vi "Read Image on Button.vi"(4 "Save in temp directory?":bool=TRUE, 6 "Append Name?":bool, 9 "image item":i32, 11 "File with Button":path) -> (0 "error out":errorcluster, 3 "png file out":path)   [LabVIEW 2021]
doc: "This example VI was obtained from this post. This strips out the saving profile and just reads the image on an existing button.\n\nhttps://forums.ni.com/t5/LabVIEW-APIs-Discussions/Set-TRUE-FALSE-Image-of-a-boolean-control-automatically-using/m-p/3419083/highlight/true#M868\n\n<b>WARNING</b>\nThis VI uses a dll call to the resource file for a LabVIEW VI/CTL - it is searching the binary data for the PNG images that the VI or CTL contains\n\n<b>Code Developed By:</b>\nTechnology Service Corporation\n1983 S Liberty Drive\nBloomington, IN 47403\nPhone: 812 558-7100\nwww.tsc.com/atcs\n\nDeveloper:\nDaniel Coons"
panel:
  out "binary PNG Data":string
  out "Resources":string[](array[string])
  # "For DEBUG"
  # "MNGI resources are 6 images\non buttons (pressed, hover, etc)\n\n-When set to a \"decal\", it should\nbe the only one"
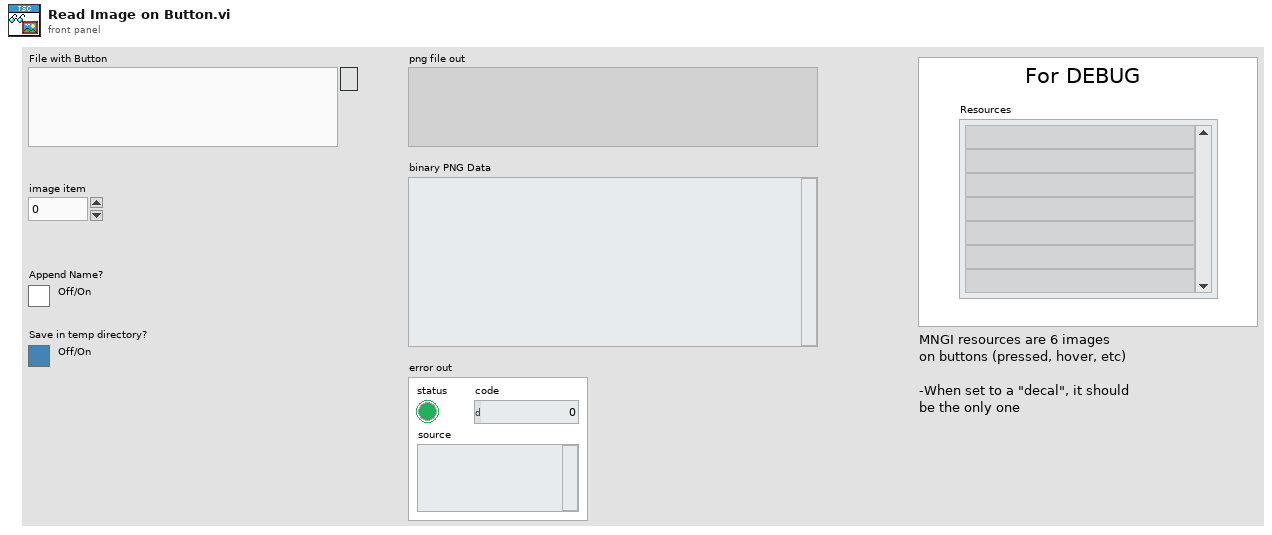
[diagram p1: front panel]
types:
  T1 = cluster{"type":u32, "id":i32, "name":string, "binary data":string}[]
  T2 = cluster{"type":u32, "id":i32, "name":string, "binary data":string}
  T3 = enum16{"open", "replace", "create", "open or create", "replace or create", "replace or create with confirmation"}
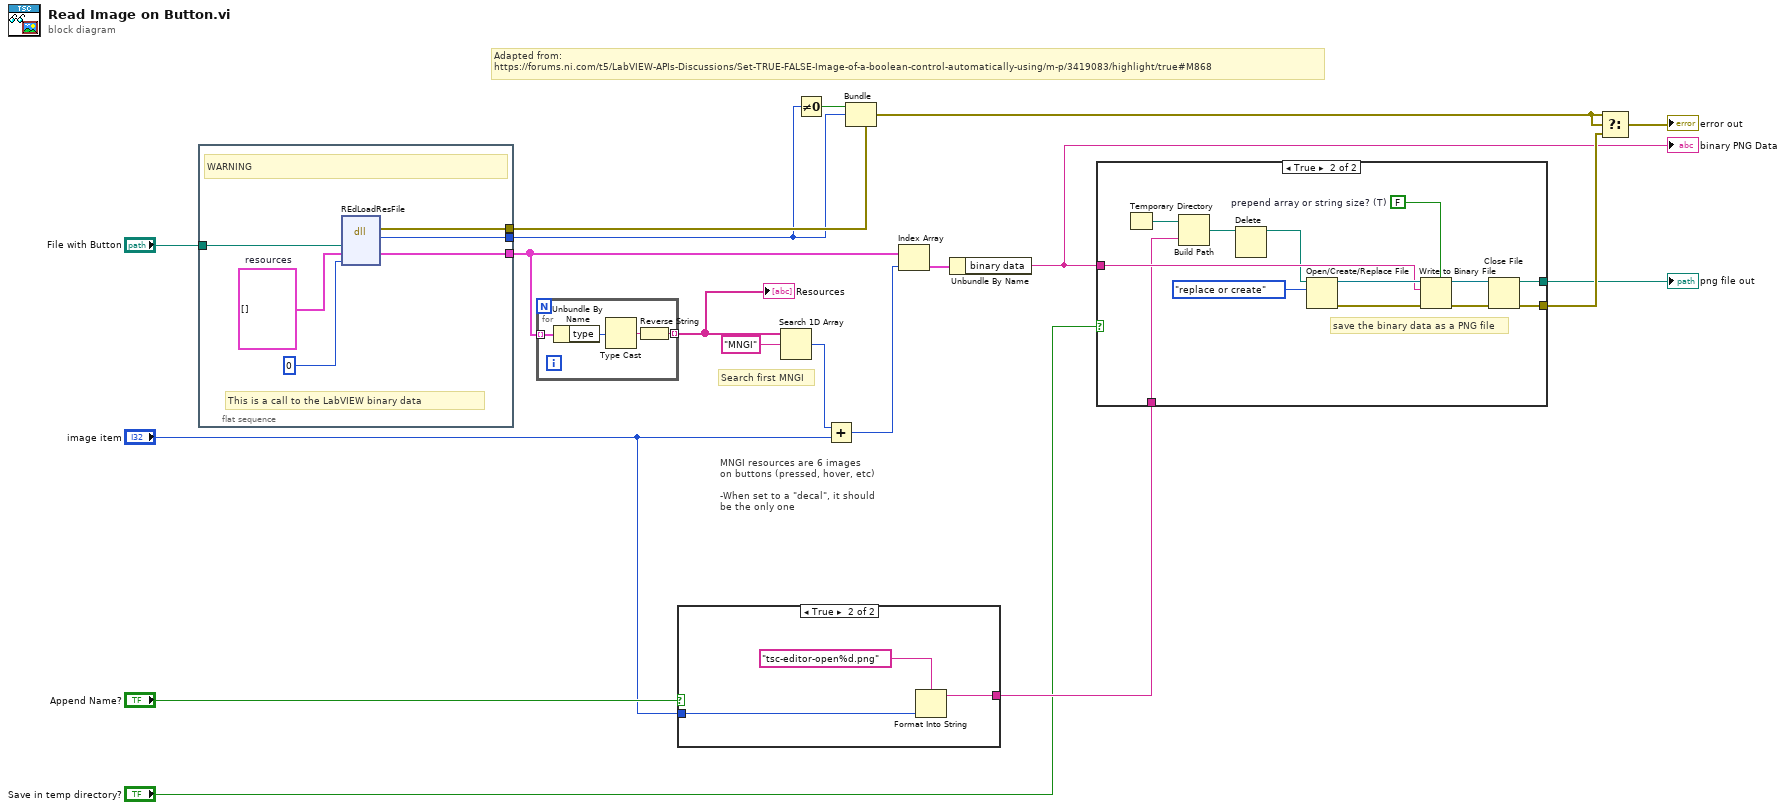
[diagram p0: block diagram]
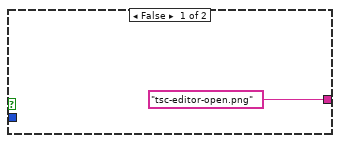
[diagram p3: hidden frame]
diagram:
  # "MNGI resources are 6 images\non buttons (pressed, hover, etc)\n\n-When set to a \"decal\", it should\nbe the only one"
  # "Adapted from:\nhttps://forums.ni.com/t5/LabVIEW-APIs-Discussions/Set-TRUE-FALSE-Image-of-a-boolean-control-automatically-using/m-p/3419083/highlight/true#M868"
  # "Search first MNGI"
  n1 = flat-sequence {
    tunnel: [w23] -> w19
    tunnel: [w22] -> w17
    tunnel: "File with Button" -> [w21]
    tunnel: [w20] -> w13
    frame #0 {
      w25 = T1 []  # resources
      # "This is a call to the LabVIEW binary data"
      # "WARNING"
      n2 = dll-call lib="LabVIEW" fn="REdLoadResFile"("path"=w21, "resources"=w25, "type"=0) -> (error out=w23:errorcluster, "return type"=w22:i32, "resources"=w20:T1)  [unwired: 3 in, 3 out]
    }
  }
  n3 = for {
    tunnel: w13 -> [w29] mode=indexing
    tunnel: [w26] -> w6 mode=indexing
    n4 = Unbundle By Name(w29) -> ("type"=w27:u32)
    n5 = Type Cast(x=w27) -> (*(type *) &x=w28:string)  [unwired: 1 out]
    n6 = Reverse String(1:w28) -> (0:w26:string)
  }
  "Resources" <- w6
  n7 = case shown="True" "Append Name?" {
    tunnel: ["tsc-editor-open.png" w32] -> w4
    tunnel: "image item" -> [_ w31]
    frame False {
    }
    frame True {
      n8 = Format Into String(format string="tsc-editor-open%d.png", w31) -> (resulting string=w32:string)  [unwired: 2 in, 1 out]
    }
  }
  n9 = Search 1D Array(1D array=w6, element="MNGI") -> (index of element=w11:i32)  [unwired: 1 out]
  n10 = Not Equal To 0?(x=w17) -> (x != 0?=w18:bool)
  n11 = Add(x=w11, y="image item") -> (x+y=w12:i32)
  n12 = Bundle(cluster=w19, "status"=w18, "code"=w17) -> (w15:errorcluster)  [unwired: 1 out]
  n13 = Index Array(array=w13, index=w12) -> (element=w10:T2)
  n14 = Unbundle By Name(w10) -> ("binary data"=w1:string)
  "binary PNG Data" <- w1
  n15 = case shown="True" "Save in temp directory?" {
    tunnel: w1 -> [_ w41]
    tunnel: [_ w38] -> w9
    tunnel: [_ w37] -> w8
    tunnel: w4 -> [_ w34]
    frame False {
    }
    frame True {
      w35 = FALSE  # prepend array or string size? (T)
      # "save the binary data as a PNG file"
      n16 = Temporary Directory() -> (w46:path)
      n17 = Build Path(base path=w46, name or relative path=w34) -> (appended path=w45:path)
      n18 = Delete(path (use dialog)=w45) -> (deleted path=w36:path)  [unwired: 4 in, 2 out]
      n19 = Open/Create/Replace File(file path (use dialog)=w36, operation (0:open)=T3."replace or create") -> (refnum out=w42:refnum<file>, error out=w43:errorcluster)  [unwired: 4 in, 1 out]
      n20 = Write to Binary File(file (use dialog)=w42, data=w41, error in=w43, 5:w35) -> (refnum out=w39:refnum<file>, error out=w40:errorcluster)  [unwired: 2 in, 1 out]
      n21 = Close File(refnum=w39, error in=w40) -> (path=w37:path, error out=w38:errorcluster)
    }
  }
  "png file out" <- w8
  n22 = Select(t=w15, s=w15, f=w9) -> (s? t:f=→"error out":errorcluster)
